vi "PQ Unit Tests.vi"() -> ()   [LabVIEW 2019]
uses:
  src/LV-Data.PG/LV-Data.PGSQL.lvclass
  src/LV-Data.PG/Typedefs/Datatypes--combo.ctl
  src/LV-Data.PG/API/Write Variable (one-row).vi
  src/LV-Data.PG/API/Write Variable (multirow).vi
  <userlib>/_OpenG.lib/array/array.llb/Delete Elements from 1D Array (DBL)__ogtk.vi
panel:
  out "Waveform Graph":dbl[][](graph)
  out "SQL":string
  out "Numeric":i32
  out "is there one more table?":bool
  out "Status":string
  out "Table":string[][](table)
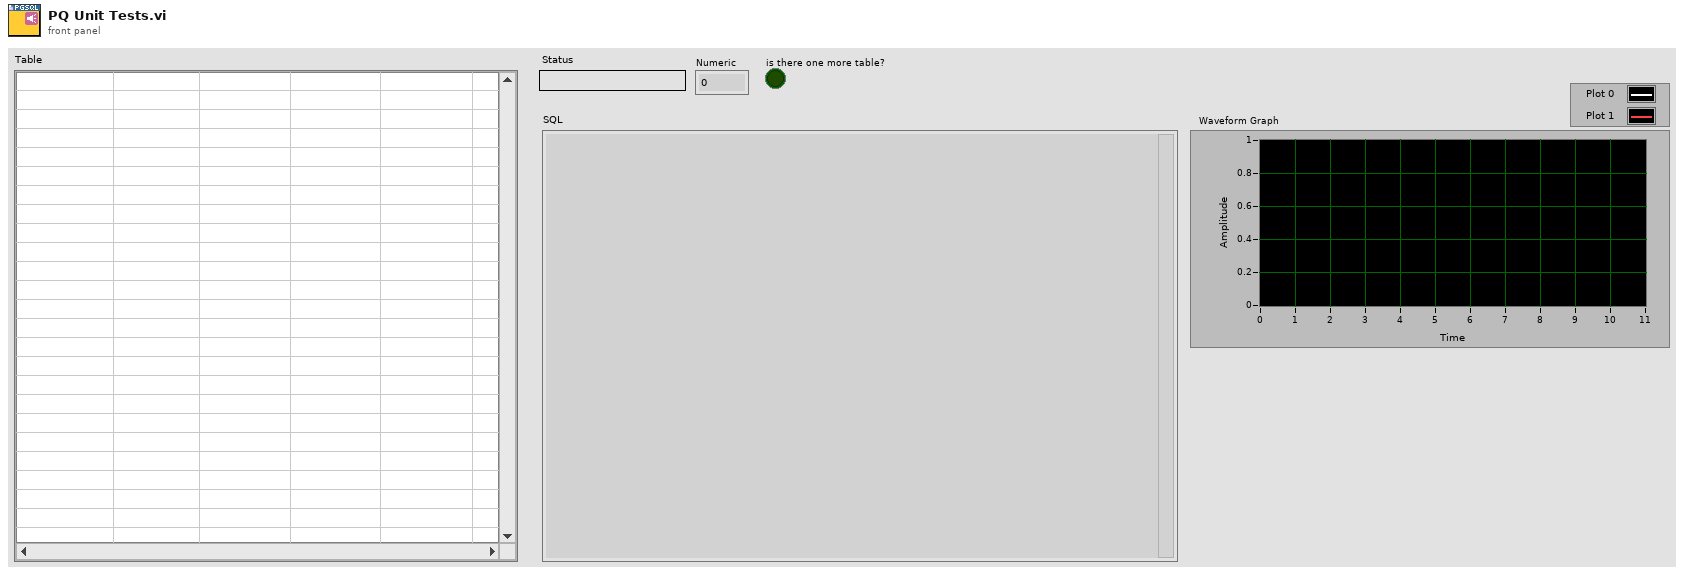
[diagram p1: front panel]
types:
  T1 = enum16{"max points", "1 second", "5 seconds", "10 seconds", "30 seconds", "1 minute", "5 minutes", "10 minutes", "30 minutes", "1 hour", "5 hours", "10 hours", "30 hours"}
  T2 = typedef "LV-Data.PGSQL.lvclass/Datatypes--combo.ctl" = string
  T3 = cluster{"integer":i32, "float":dbl, "string":string, "boolean":bool}
  T4 = cluster{"integer":i32, "float":dbl, "string":string, "boolean":bool}[]
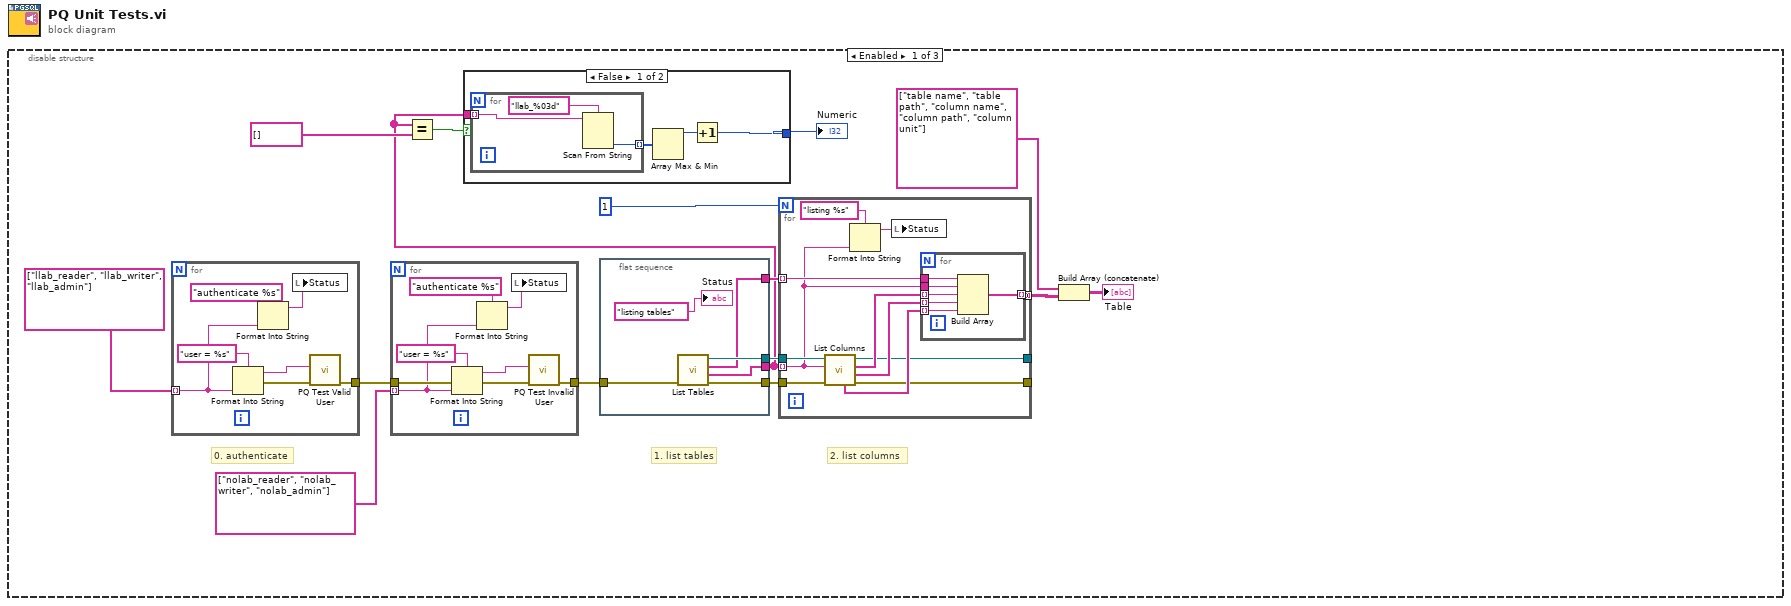
[diagram p0: block diagram]
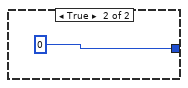
[diagram p2: hidden frame]
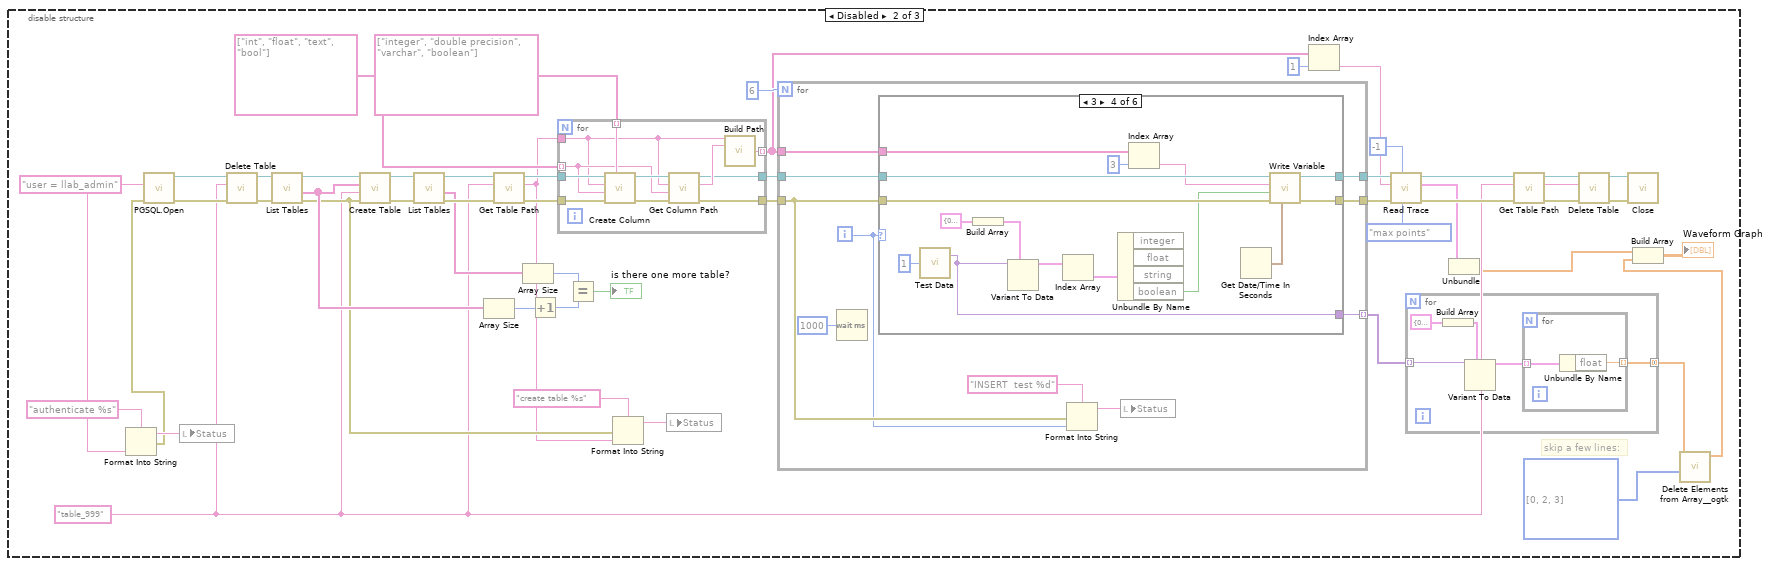
[diagram p3: hidden frame]
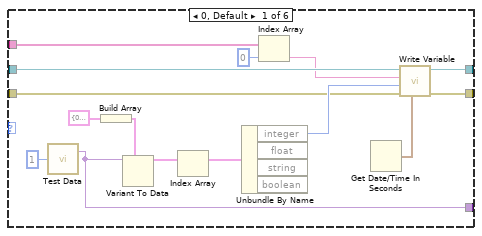
[diagram p4: hidden frame]
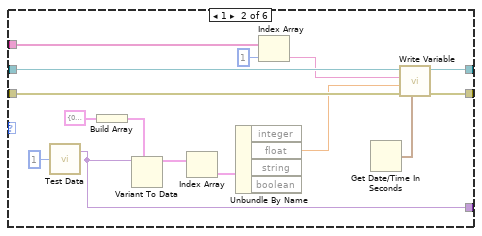
[diagram p5: hidden frame]
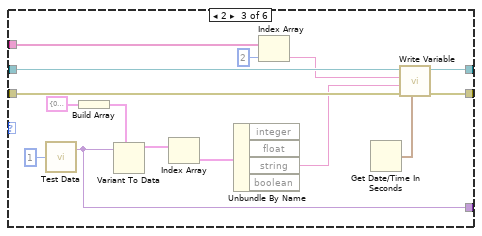
[diagram p6: hidden frame]
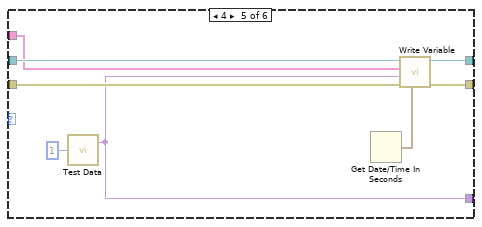
[diagram p7: hidden frame]
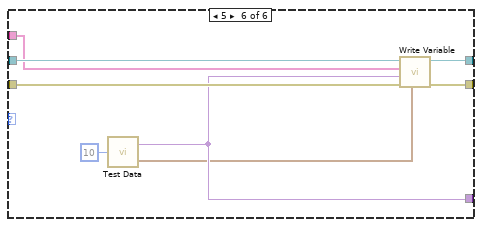
[diagram p8: hidden frame]
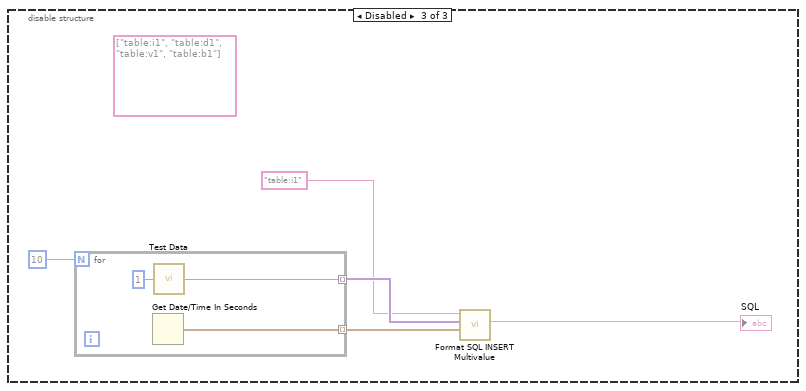
[diagram p9: hidden frame]
diagram:
  n1 = disable-structure "Diagram Disable Structure" shown="Enabled" {
    frame Enabled {
      # "0. authenticate"
      # "2. list columns"
      # "1. list tables"
      n2 = for {
        tunnel: [w38] -> w3
        tunnel: string[] ["llab_reader", "llab_writer", "llab_admin"] -> [w41] mode=indexing
        n3 = Format Into String(format string="user = %s" ("Connection String"), w41) -> (resulting string=w39:string, error out=w40:errorcluster)  [unwired: 2 in]
        n4 = Format Into String(format string="authenticate %s", w41) -> (resulting string=w43:string)  [unwired: 2 in, 1 out]
        n5 = local write "Status"(w43) -> ()
        n6 = call "PQ Test Valid User.vi"("error in (no error)"=w40, "Connection String"=w39) -> ("error out"=w38:errorcluster)  [unwired: 9 in]
      }
      n7 = for {
        tunnel: [w18] -> w1
        tunnel: w3 -> [w17]
        tunnel: string[] ["nolab_reader", "nolab_writer", "nolab_admin"] -> [w16] mode=indexing
        n8 = Format Into String(format string="user = %s" ("Connection String"), error in=w17, w16) -> (resulting string=w19:string, error out=w20:errorcluster)  [unwired: 1 in]
        n9 = Format Into String(format string="authenticate %s", w16) -> (resulting string=w22:string)  [unwired: 2 in, 1 out]
        n10 = local write "Status"(w22) -> ()
        n11 = call "PQ Test Invalid User.vi"("error in (no error)"=w20, "Connection String"=w19) -> ("error out"=w18:errorcluster)  [unwired: 9 in]
      }
      n12 = Equal?(x=w4, y=string[] []) -> (x = y?=w6:bool)
      n13 = case shown="False" w6 {
        tunnel: w4 -> [w33 _]
        tunnel: [w30 0] -> w5
        frame False {
          n14 = for {
            tunnel: w33 -> [w35] mode=indexing
            tunnel: [w34] -> w32 mode=indexing
            n15 = Scan From String(format string="llab_%03d", input string=w35) -> (output 1=w34:i32)  [unwired: 3 in, 3 out]
          }
          n16 = Array Max & Min(array=w32) -> (max value=w31:i32)  [unwired: 3 out]
          n17 = Increment(x=w31) -> (x+1=w30:i32)
        }
        frame True {
        }
      }
      "Numeric" <- w5
      n18 = flat-sequence {
        tunnel: [w29] -> w15
        tunnel: [w28] -> w14
        tunnel: [w27] -> w4
        tunnel: [w26] -> w13
        tunnel: w1 -> [w24]
        frame #0 {
          n19 = call "List Tables.vi"("error in (no error)"=w24) -> ("error out"=w28:errorcluster, "Table Paths"=w27:string[], "Table Names"=w26:string[], "Data.PG"=w29:refnum<class "LV-Data.PGSQL.lvclass">)  [unwired: 7 in]
          "Status" <- "listing tables"
        }
      }
      n20 = for {
        N: 1 -> [_]
        tunnel: w15 -> [w56]
        tunnel: w14 -> [w55]
        tunnel: w4 -> [w47] mode=indexing
        tunnel: w13 -> [w50] mode=indexing
        tunnel: [w53] -> w11 mode=concatenating
        tunnel: [w46] -> _
        tunnel: [w45] -> _
        n21 = call "List Columns.vi"("error in (no error)"=w55, "Table Path"=w47, "Data.PG"=w56) -> ("error out"=w46:errorcluster, "Column Paths"=w51:string[], "Column Names"=w52:string[], "Data.PG out"=w45:refnum<class "LV-Data.PGSQL.lvclass">, "Column Units"=w54:string[])  [unwired: 4 in]
        n22 = Format Into String(format string="listing %s", w47) -> (resulting string=w48:string)  [unwired: 2 in, 1 out]
        n23 = local write "Status"(w48) -> ()
        n24 = for {
          tunnel: w50 -> [w62]
          tunnel: w52 -> [w61] mode=indexing
          tunnel: w51 -> [w60] mode=indexing
          tunnel: w54 -> [w59] mode=indexing
          tunnel: [w58] -> w53 mode=indexing
          tunnel: w47 -> [w57]
          n25 = Build Array(w62, w57, w61, w60, w59) -> (w58:string[])
        }
      }
      n26 = Build Array (concatenate)(string[] ["table name", "table path", "column name", "column path", "column unit"] ("appended array"), w11) -> (→"Table":string[][])
    }
    frame Disabled {
      w75 = "table_999" ("Table Path")
      w85 = "user = llab_admin" ("Connection String")
      # "skip a few lines:"
      n27 = Format Into String(format string="authenticate %s", w85) -> (resulting string=w87:string, error out=w84:errorcluster)  [unwired: 2 in]
      n28 = call "PGSQL.Open.vi"("error in (no error)"=w84, "Connection String"=w85) -> ("error out"=w114:errorcluster, "Data.PG out"=w113:refnum<class "LV-Data.PGSQL.lvclass">)  [unwired: 8 in]
      n29 = local write "Status"(w87) -> ()
      n30 = call "Delete Table.vi"("error in"=w114, "Table Path"=w75, "LV-Data.PGSQL"=w113) -> ("error out"=w102:errorcluster, "LV-Data.PGSQL out"=w101:refnum<class "LV-Data.PGSQL.lvclass">)  [unwired: 7 in]
      n31 = call "List Tables.vi"("error in (no error)"=w102, "Data.PG"=w101) -> ("error out"=w81:errorcluster, "Table Paths"=w106:string[], "Data.PG"=w103:refnum<class "LV-Data.PGSQL.lvclass">)  [unwired: 6 in, 1 out]
      n32 = call "Create Table.vi"("error in (no error)"=w81, "New Table Name"=w75, "Table Paths"=w106, "Data.PGSQL"=w103) -> ("error out"=w104:errorcluster, "Data.PGSQL out"=w105:refnum<class "LV-Data.PGSQL.lvclass">)  [unwired: 6 in]
      n33 = call "List Tables.vi"("error in (no error)"=w104, "Data.PG"=w105) -> ("error out"=w100:errorcluster, "Table Paths"=w88:string[], "Data.PG"=w99:refnum<class "LV-Data.PGSQL.lvclass">)  [unwired: 6 in, 1 out]
      n34 = Array Size(array=w106) -> (size(s)=w107:i32)
      n35 = call "Get Table Path.vi"("error in (no error)"=w100, "Table Name"=w75, "Data.PG"=w99) -> ("error out"=w97:errorcluster, "Table Path"=w80:string, "Data.PG out"=w98:refnum<class "LV-Data.PGSQL.lvclass">)  [unwired: 5 in, 1 out]
      n36 = Array Size(array=w88) -> (size(s)=w108:i32)
      n37 = Increment(x=w107) -> (x+1=w109:i32)
      n38 = for {
        tunnel: w80 -> [w212]
        tunnel: w98 -> [w218]
        tunnel: w97 -> [w217]
        tunnel: T2[] ["integer", "double precision", "varchar", "boolean"] ("Array") -> [w216] mode=indexing
        tunnel: string[] ["int", "float", "text", "bool"] -> [w213] mode=indexing
        tunnel: [w210] -> w94
        tunnel: [w209] -> w92
        tunnel: [w208] -> w73 mode=indexing
        n39 = call "Create Column.vi"("Data type"=w216, "error in (no error)"=w217, "new column name"=w213, "selected table path"=w212, "Data.PGSQL in"=w218) -> ("error out"=w215:errorcluster, "Data.PGSQL out"=w214:refnum<class "LV-Data.PGSQL.lvclass">)  [unwired: 5 in]
        n40 = call "Get Column Path.vi"("error in (no error)"=w215, "Column Name"=w213, "Table path"=w212, "Data.PG in"=w214) -> ("error out"=w209:errorcluster, "Column Path"=w211:string, "Data.PG out"=w210:refnum<class "LV-Data.PGSQL.lvclass">)  [unwired: 4 in, 1 out]
        n41 = call "Build Path.vi"("Table path"=w212, "Column path"=w211) -> ("PG path"=w208:string)  [unwired: 13 in]
      }
      n42 = Equal?(x=w108, y=w109) -> (x = y?=→"is there one more table?":bool)
      n43 = Format Into String(format string="create table %s", error in=w81, w80) -> (resulting string=w82:string)  [unwired: 1 in, 1 out]
      n44 = local write "Status"(w82) -> ()
      n45 = for {
        N: 6 -> [_]
        tunnel: w73 -> [w131]
        tunnel: w94 -> [w130]
        tunnel: [w129] -> w79
        tunnel: [w128] -> w77
        tunnel: w92 -> [w124]
        tunnel: [w122] -> w70 mode=indexing
        i -> [w123]
        n46 = Wait (ms)(milliseconds to wait=u32 1000) -> ()  [unwired: 1 out]
        n47 = case shown="3" w123 {
          tunnel: w131 -> [w140 w157 w172 w187 w195 w205]
          tunnel: w130 -> [w146 w161 w176 w191 w199 w207]
          tunnel: [w143 w158 w173 w188 w196 w206] -> w129
          tunnel: [w135 w153 w168 w183 w193 w203] -> w128
          tunnel: w124 -> [w136 w154 w169 w184 w194 w204]
          tunnel: [w132 w147 w162 w177 w192 w202] -> w122
          frame 0, Default {
            n48 = call "Test Data.vi"("Size"=1) -> ("Data"=w132:variant)  [unwired: 1 out]
            n49 = Build Array(T3 {"integer"=0, "float"=0.0, "string"="", "boolean"=TRUE} ("cluster")) -> (w134:T4)
            n50 = Variant To Data(type=w134, Variant=w132) -> (data=w142:T4)  [unwired: 1 in, 1 out]
            n51 = Index Array(array=w142) -> (element=w133:T3)  [unwired: 1 in]
            n52 = Unbundle By Name(w133) -> ("integer"=w138:i32)  [unwired: 3 out]
            n53 = Index Array(array=w140, index=0) -> (element=w139:string)
            n54 = Get Date/Time In Seconds() -> (seconds since 1Jan1904=w144:timestamp)
            n55 = call-poly "Write Variable.vi"("Time Stamp"=w144, "error in (no error)"=w136, "Data"=w138, "variable"=w139, "Data.PG in"=w146) -> ("error out"=w135:errorcluster, "Data.PG out"=w143:refnum<class "LV-Data.PGSQL.lvclass">)  [unwired: 3 in, 2 out]
          }
          frame 1 {
            n56 = call "Test Data.vi"("Size"=1) -> ("Data"=w147:variant)  [unwired: 1 out]
            n57 = Build Array(T3 {"integer"=0, "float"=0.0, "string"="", "boolean"=TRUE} ("cluster")) -> (w149:T4)
            n58 = Variant To Data(type=w149, Variant=w147) -> (data=w151:T4)  [unwired: 1 in, 1 out]
            n59 = Index Array(array=w151) -> (element=w148:T3)  [unwired: 1 in]
            n60 = Unbundle By Name(w148) -> ("float"=w152:dbl)  [unwired: 3 out]
            n61 = Index Array(array=w157, index=1) -> (element=w156:string)
            n62 = Get Date/Time In Seconds() -> (seconds since 1Jan1904=w159:timestamp)
            n63 = call-poly "Write Variable.vi"("Time Stamp"=w159, "error in (no error)"=w154, "Data"=w152, "variable"=w156, "Data.PG in"=w161) -> ("error out"=w153:errorcluster, "Data.PG out"=w158:refnum<class "LV-Data.PGSQL.lvclass">)  [unwired: 3 in, 2 out]
          }
          frame 2 {
            n64 = call "Test Data.vi"("Size"=1) -> ("Data"=w162:variant)  [unwired: 1 out]
            n65 = Build Array(T3 {"integer"=0, "float"=0.0, "string"="", "boolean"=TRUE} ("cluster")) -> (w164:T4)
            n66 = Variant To Data(type=w164, Variant=w162) -> (data=w166:T4)  [unwired: 1 in, 1 out]
            n67 = Index Array(array=w166) -> (element=w163:T3)  [unwired: 1 in]
            n68 = Unbundle By Name(w163) -> ("string"=w167:string)  [unwired: 3 out]
            n69 = Index Array(array=w172, index=2) -> (element=w171:string)
            n70 = Get Date/Time In Seconds() -> (seconds since 1Jan1904=w174:timestamp)
            n71 = call-poly "Write Variable.vi"("Time Stamp"=w174, "error in (no error)"=w169, "Data"=w167, "variable"=w171, "Data.PG in"=w176) -> ("error out"=w168:errorcluster, "Data.PG out"=w173:refnum<class "LV-Data.PGSQL.lvclass">)  [unwired: 3 in, 2 out]
          }
          frame 3 {
            n72 = call "Test Data.vi"("Size"=1) -> ("Data"=w177:variant)  [unwired: 1 out]
            n73 = Build Array(T3 {"integer"=0, "float"=0.0, "string"="", "boolean"=TRUE} ("cluster")) -> (w179:T4)
            n74 = Variant To Data(type=w179, Variant=w177) -> (data=w181:T4)  [unwired: 1 in, 1 out]
            n75 = Index Array(array=w181) -> (element=w178:T3)  [unwired: 1 in]
            n76 = Unbundle By Name(w178) -> ("boolean"=w182:bool)  [unwired: 3 out]
            n77 = Index Array(array=w187, index=3) -> (element=w186:string)
            n78 = Get Date/Time In Seconds() -> (seconds since 1Jan1904=w189:timestamp)
            n79 = call-poly "Write Variable.vi"("Time Stamp"=w189, "error in (no error)"=w184, "Data"=w182, "variable"=w186, "Data.PG in"=w191) -> ("error out"=w183:errorcluster, "Data.PG out"=w188:refnum<class "LV-Data.PGSQL.lvclass">)  [unwired: 3 in, 2 out]
          }
          frame 4 {
            n80 = call "Test Data.vi"("Size"=1) -> ("Data"=w192:variant)  [unwired: 1 out]
            n81 = Get Date/Time In Seconds() -> (seconds since 1Jan1904=w197:timestamp)
            n82 = call-poly "Write Variable.vi"("Time Stamp"=w197, "error in (no error)"=w194, "Data"=w192, "variable"=w195, "Data.PG in"=w199) -> ("error out"=w193:errorcluster, "Data.PG out"=w196:refnum<class "LV-Data.PGSQL.lvclass">)  [unwired: 3 in, 2 out]
          }
          frame 5 {
            n83 = call "Test Data.vi"("Size"=10) -> ("Data"=w202:variant, "Timestamps"=w200:timestamp[])
            n84 = call-poly "Write Variable.vi"("Time Stamps"=w200, "error in (no error)"=w204, "Data"=w202, "Path(s)"=w205, "Data.PG in"=w207) -> ("error out"=w203:errorcluster, "Data.PG out"=w206:refnum<class "LV-Data.PGSQL.lvclass">)  [unwired: 3 in, 2 out]
          }
        }
        n85 = Format Into String(format string="INSERT  test %d", error in=w124, w123) -> (resulting string=w126:string)  [unwired: 1 in, 1 out]
        n86 = local write "Status"(w126) -> ()
      }
      n87 = Index Array(array=w73, index=1) -> (element=w72:string)
      n88 = call "Read Trace.vi"("time_bucket"=T1."max points", "max points (-1 = all)"=-1, "error in (no error)"=w77, "PG path"=w72, "Data.PGQL in"=w79) -> ("error out"=w76:errorcluster, "Trace"=w71:cluster{timestamp[], dbl[]}, "Data.PGSQL out"=w78:refnum<class "LV-Data.PGSQL.lvclass">)  [unwired: 2 in, 2 out]
      n89 = for {
        tunnel: w70 -> [w116] mode=indexing
        tunnel: [w115] -> w68 mode=concatenating
        n90 = Build Array(T3 {"integer"=0, "float"=0.0, "string"="", "boolean"=TRUE} ("cluster")) -> (w118:T4)
        n91 = Variant To Data(type=w118, Variant=w116) -> (data=w117:T4)  [unwired: 1 in, 1 out]
        n92 = for {
          tunnel: w117 -> [w121] mode=indexing
          tunnel: [w120] -> w115 mode=indexing
          n93 = Unbundle By Name(w121) -> ("float"=w120:dbl)
        }
      }
      n94 = Unbundle(w71) -> (w63:dbl[])  [unwired: 1 out]
      n95 = call "Get Table Path.vi"("error in (no error)"=w76, "Table Name"=w75, "Data.PG"=w78) -> ("error out"=w91:errorcluster, "Table Path"=w89:string, "Data.PG out"=w90:refnum<class "LV-Data.PGSQL.lvclass">)  [unwired: 5 in, 1 out]
      n96 = call "Delete Table.vi"("error in"=w91, "Table Path"=w89, "LV-Data.PGSQL"=w90) -> ("error out"=w112:errorcluster, "LV-Data.PGSQL out"=w111:refnum<class "LV-Data.PGSQL.lvclass">)  [unwired: 7 in]
      n97 = call-dynamic "Close.vi"("error in (no error)"=w112, "Data.PG in"=w111) -> ()  [unwired: 8 in, 2 out]
      n98 = call-poly <userlib>:"Delete Elements from Array__ogtk.vi"("indices"=i32[] [0, 2, 3], "array"=w68) -> ("array w/ subset deleted"=w67:dbl[])  [unwired: 8 in, 1 out]
      n99 = Build Array(w63, w67) -> (→"Waveform Graph":dbl[][])
    }
    frame Disabled {
      (unwired) string[] ["table:i1", "table:d1", "table:v1", "table:b1"]
      n100 = for {
        N: 10 -> [_]
        tunnel: [w225] -> w222 mode=indexing
        tunnel: [w224] -> w221 mode=indexing
        n101 = Get Date/Time In Seconds() -> (seconds since 1Jan1904=w224:timestamp)
        n102 = call "Test Data.vi"("Size"=1) -> ("Data"=w225:variant)
      }
      n103 = call "Format SQL INSERT Multivalue.vi"("Data"=w221, "Path(s)"=w222, "Data.PG in"="table:i1" ("String")) -> ("SQL"=→"SQL":string)  [unwired: 5 in, 3 out]
    }
  }
